vi "Static Demo.vi"() -> ()   [LabVIEW 2020]
uses:
  <extravilib>/ChannelInstances/Flex-c(dbl,dbl,a[.](dbl)).lvlib
  <extravilib>/ChannelInstances/Flex-dbl.lvlib
  FlexBlocks/FlexBlocks.lvlib
  FlexBlocks/Command.ctl
  FlexBlocks/Run Action.ctl
  FlexBlocks/Block State.ctl
  FlexBlocks/Block Status.ctl
  FlexBlocks/Block Status with Error.ctl
  <extravilib>/ChannelInstances/Flex-t'Function Generator.lvlib-Shape.ctl'.lvlib
  FlexBlocks/Shape.ctl
  Workers/Function Generator/Function Generator.lvlib
panel:
  out "Usage Ratio":dbl[](array[slide]) scale=0.0..1.0
  out "Queued Count":i32[](array[numeric])
  out "Sequence":u32
  in  "Read Delay":u32(slide) scale=0.0..1000.0
  out "Status":T1={"Status"={"State"=enum."Stop", "i"=217, "Init"=TRUE, "Started"=TRUE, "Action"=enum."N/A"}, "Error"={"status"=FALSE, "code"=0, "source"=""}}
  in  "Send":bool
  in  "Command":T5=enum."Run"
  in  "stop":bool
  in  "Shape":T6
  in  "Offset":dbl(slide) scale=-5.0..5.0
  in  "Phase":dbl(slide)=0.602006688963229 scale=-180.0..180.0
  in  "Amplitude":dbl(slide)=2.508361204013378 scale=0.0..5.0
  in  "Frequency":dbl(slide)=24.926421404682273 scale=1.0..50.0
  out "Graph":cluster{"t0":dbl, "dt":dbl, "y":dbl[]}(graph)
  # "Buffer Playground"
  # "Manager Sim"
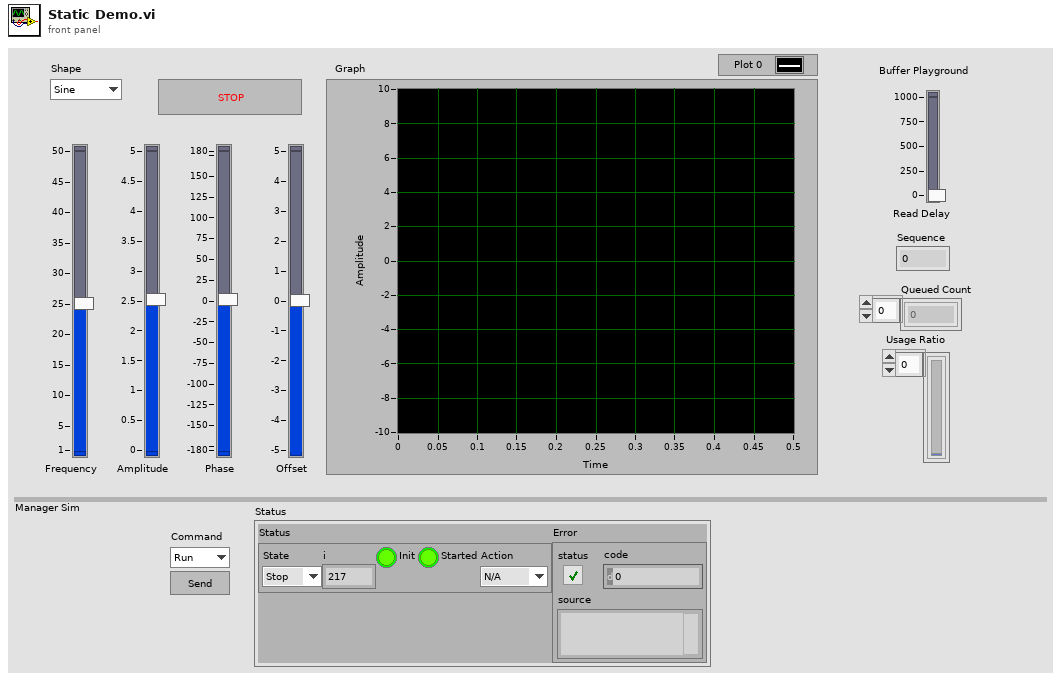
[diagram p1: front panel]
types:
  T1 = typedef "FlexBlocks.lvlib/Block Status with Error.ctl" = cluster{"Status":T2, "Error":errorcluster}
  T2 = typedef "FlexBlocks.lvlib/Block Status.ctl" = cluster{"State":T3, "i":i32, "Init":bool, "Started":bool, "Action":T4}
  T3 = typedef "FlexBlocks.lvlib/Block State.ctl" = enum16{"Idle", "Init", "Start", "Run", "Stop"}
  T4 = typedef "FlexBlocks.lvlib/Run Action.ctl" = enum16{"N/A", "Read", "Work", "Write"}
  T5 = typedef "FlexBlocks.lvlib/Command.ctl" = enum16{"Close", "Step", "Run", "Pause", "Init"}
  T6 = typedef "Function Generator.lvlib/Shape.ctl" = enum16{"Sine", "Square", "Triangle", "Saw"}
  T7 = typedef "Flex-t'Function Generator.lvlib-Shape.ctl'.lvlib/))Channel.ctl" = refnum<queue>
  T8 = typedef "Flex-dbl.lvlib/))Channel.ctl" = refnum<queue>
  T9 = typedef "Flex-c(dbl,dbl,a[.](dbl)).lvlib/))Channel.ctl" = refnum<queue>
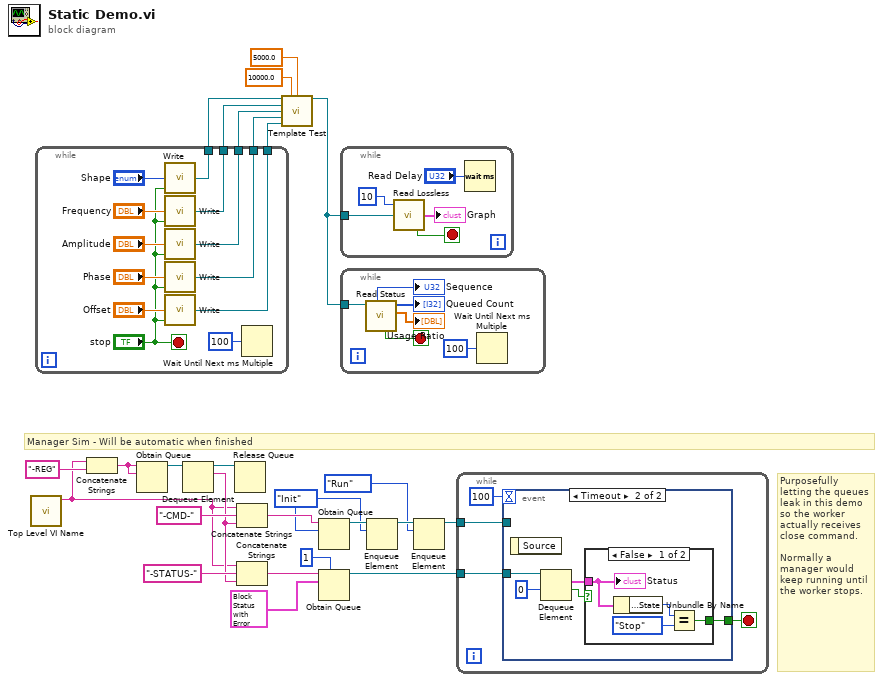
[diagram p0: block diagram]
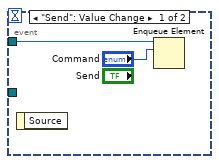
[diagram p2: hidden frame]
diagram:
  w5 = Command."Init" ("Command")
  # "Purposefully letting the queues leak in this demo so the worker actually receives close command.\n\nNormally a manager would keep running until the worker stops."
  # "Manager Sim - Will be automatic when finished"
  n1 = call "Top Level VI Name.vi"() -> ("Top Level VI Name"=w8:string)  [unwired: 11 in]
  n2 = while {
    tunnel: [w38] -> w26
    tunnel: [w37] -> w23
    tunnel: [w36] -> w22
    tunnel: [w35] -> w21
    tunnel: [w29] -> w1
    stop <- "stop" stop-if-true
    n3 = call <extravilib>:"Write.vi"("element"="Shape", "Close? (F)"="stop") -> ("channel"=w29:T7)  [unwired: 3 in, 2 out]
    n4 = call <extravilib>:"Write.vi"("element"="Frequency", "Close? (F)"="stop") -> ("channel"=w35:T8)  [unwired: 3 in, 2 out]
    n5 = call <extravilib>:"Write.vi"("element"="Amplitude", "Close? (F)"="stop") -> ("channel"=w36:T8)  [unwired: 3 in, 2 out]
    n6 = call <extravilib>:"Write.vi"("element"="Phase", "Close? (F)"="stop") -> ("channel"=w37:T8)  [unwired: 3 in, 2 out]
    n7 = call <extravilib>:"Write.vi"("element"="Offset", "Close? (F)"="stop") -> ("channel"=w38:T8)  [unwired: 3 in, 2 out]
    n8 = Wait Until Next ms Multiple(millisecond multiple=u32 100) -> ()  [unwired: 1 out]
  }
  n9 = Concatenate Strings(w8, "-REG" ("string")) -> (w13:string)
  n10 = Obtain Queue(name (unnamed)=w13, element data type=w13) -> (queue out=w12:refnum<queue>)  [unwired: 3 in, 2 out]
  n11 = Dequeue Element(queue=w12) -> (queue out=w10:refnum<queue>, element=w11:string)  [unwired: 2 in, 2 out]
  n12 = Release Queue(queue=w10) -> ()  [unwired: 2 in, 3 out]
  n13 = Concatenate Strings(w8, "-CMD-" ("string"), w11) -> (w20:string)
  n14 = Concatenate Strings(w8, "-STATUS-" ("string"), w11) -> (w19:string)
  n15 = call "Template Test.vi"("Shape"=w1, "Sample Frequency"=10000.0, "Sample Count"=5000.0, "Frequency"=w21, "Amplitude"=w22, "Phase"=w23, "Offset"=w26) -> ("Out"=w7:T9)  [unwired: 8 in]
  n16 = Obtain Queue(name (unnamed)=w20, element data type=w5) -> (queue out=w6:refnum<queue>)  [unwired: 3 in, 2 out]
  n17 = Obtain Queue(max queue size (-1, unlimited)=1, name (unnamed)=w19, element data type=T1 {"Status"={"State"=enum."Init", "i"=0, "Init"=FALSE, "Started"=FALSE, "Action"=enum."N/A"}, "Error"={"status"=FALSE, "code"=0, "source"=""}} ("Block Status with Error")) -> (queue out=w9:refnum<queue>)  [unwired: 2 in, 2 out]
  n18 = while {
    tunnel: w7 -> [w42]
    stop <- w41 stop-if-true
    n19 = call <extravilib>:"Read Lossless.vi"("Depth (Unlimited)"=10, "FlexChannel"=w42) -> ("Element"=→"Graph":cluster{"t0":dbl, "dt":dbl, "y":dbl[]}, "Closed?"=w41:bool)  [unwired: 3 in, 1 out]
    n20 = Wait (ms)(milliseconds to wait="Read Delay") -> ()  [unwired: 1 out]
  }
  n21 = while {
    tunnel: w7 -> [w49]
    stop <- w48 stop-if-true
    n22 = call <extravilib>:"Read Status.vi"("channel"=w49) -> ("Usage Ratio"=→"Usage Ratio":dbl[], "Queued Count"=→"Queued Count":i32[], "Closed?"=w48:bool, "Sequence"=→"Sequence":u32)  [unwired: 4 in, 3 out]
    n23 = Wait Until Next ms Multiple(millisecond multiple=u32 100) -> ()  [unwired: 1 out]
  }
  n24 = Enqueue Element(queue=w6, element=w5) -> (queue out=w4:refnum<queue>)  [unwired: 2 in, 2 out]
  n25 = Enqueue Element(queue=w4, element=Command."Run" ("Command")) -> (queue out=w2:refnum<queue>)  [unwired: 2 in, 2 out]
  n26 = while {
    tunnel: w2 -> [w51]
    tunnel: w9 -> [w50]
    stop <- w53 stop-if-true
    n27 = event shown="[1] Timeout" {
      selector: _ -> [_ _]
      dyn-events: _ -> [_ _]
      timeout: 100 -> [_ _]
      tunnel: [_ w56] -> w53
      tunnel: w51 -> [w55 _]
      tunnel: w50 -> [_ w58]
      event "Send": Value Change {
        n28 = event-data() -> ()  [unwired: 1 in, 1 out]
        n29 = Enqueue Element(queue=w55, element="Command") -> ()  [unwired: 2 in, 3 out]
      }
      event Timeout {
        n30 = event-data() -> ()  [unwired: 1 in, 1 out]
        n31 = Dequeue Element(queue=w58, timeout in ms (-1)=0) -> (element=w60:T1, timed out?=w59:bool)  [unwired: 1 in, 2 out]
        n32 = case shown="False" w59 {
          tunnel: w60 -> [w64 _]
          tunnel: [w61 _] -> w56
          frame False {
            n33 = Unbundle By Name(w64) -> ("Status.State"=w63:T3)
            n34 = Equal?(x=w63, y=Block_State."Stop") -> (x = y?=w61:bool)
            "Status" <- w64
          }
          frame True {
          }
        }
      }
    }
  }
